vi "Format DescribeInstances_LVXML_ReservationSet_Loop.vi"(8 "error in (no error)":errorcluster, 11 "Siblings":T18(array[cluster])) -> (0 "error out":errorcluster, 3 "reservationSet":T1[](array[typedef]))   [LabVIEW 2014, in "AWS_EC2.lvlib" / "AWS_EC2.lvclass"]
uses:
  AWS_EC2.lvclass
  lv-xml-parser/r0/trunk/VI Source/EventType.ctl
  EC2 Datatypes/ReservationInfoType.ctl
  EC2 Datatypes/GroupItemType.ctl
  EC2 Datatypes/RunningInstancesItemsType.ctl
  EC2 Datatypes/InstanceStateType.ctl
  EC2 Datatypes/ProductCodeSetItemType.ctl
  EC2 Datatypes/PlacementResponseType.ctl
  EC2 Datatypes/GroupItemTypeSet.ctl
  EC2 Datatypes/StateReasonType.ctl
  EC2 Datatypes/InstanceBlockDeviceMappingResponseItemType.ctl
  EC2 Datatypes/EbsInstanceBlockDeviceMappingResponseType.ctl
  EC2 Datatypes/ResourceTagSetItemType.ctl
  EC2 Datatypes/InstanceNetworkInterfaceSetItemType.ctl
  EC2 Datatypes/InstanceNetworkInterfaceAttachmentType.ctl
  EC2 Datatypes/InstanceNetworkInterfaceAssociationType.ctl
  EC2 Datatypes/InstancePrivateIpAddressesSetItemType.ctl
  EC2 Datatypes/IamInstanceProfileResponseType.ctl
  lv-xml-parser/r0/trunk/VI Source/LV XML Parser.lvlib
  AWS_EC2.lvlib
panel:
  out "AWS_EC2 out":refnum<class "AWS_EC2.lvclass">
  in  "AWS_EC2 in":refnum<class "AWS_EC2.lvclass">
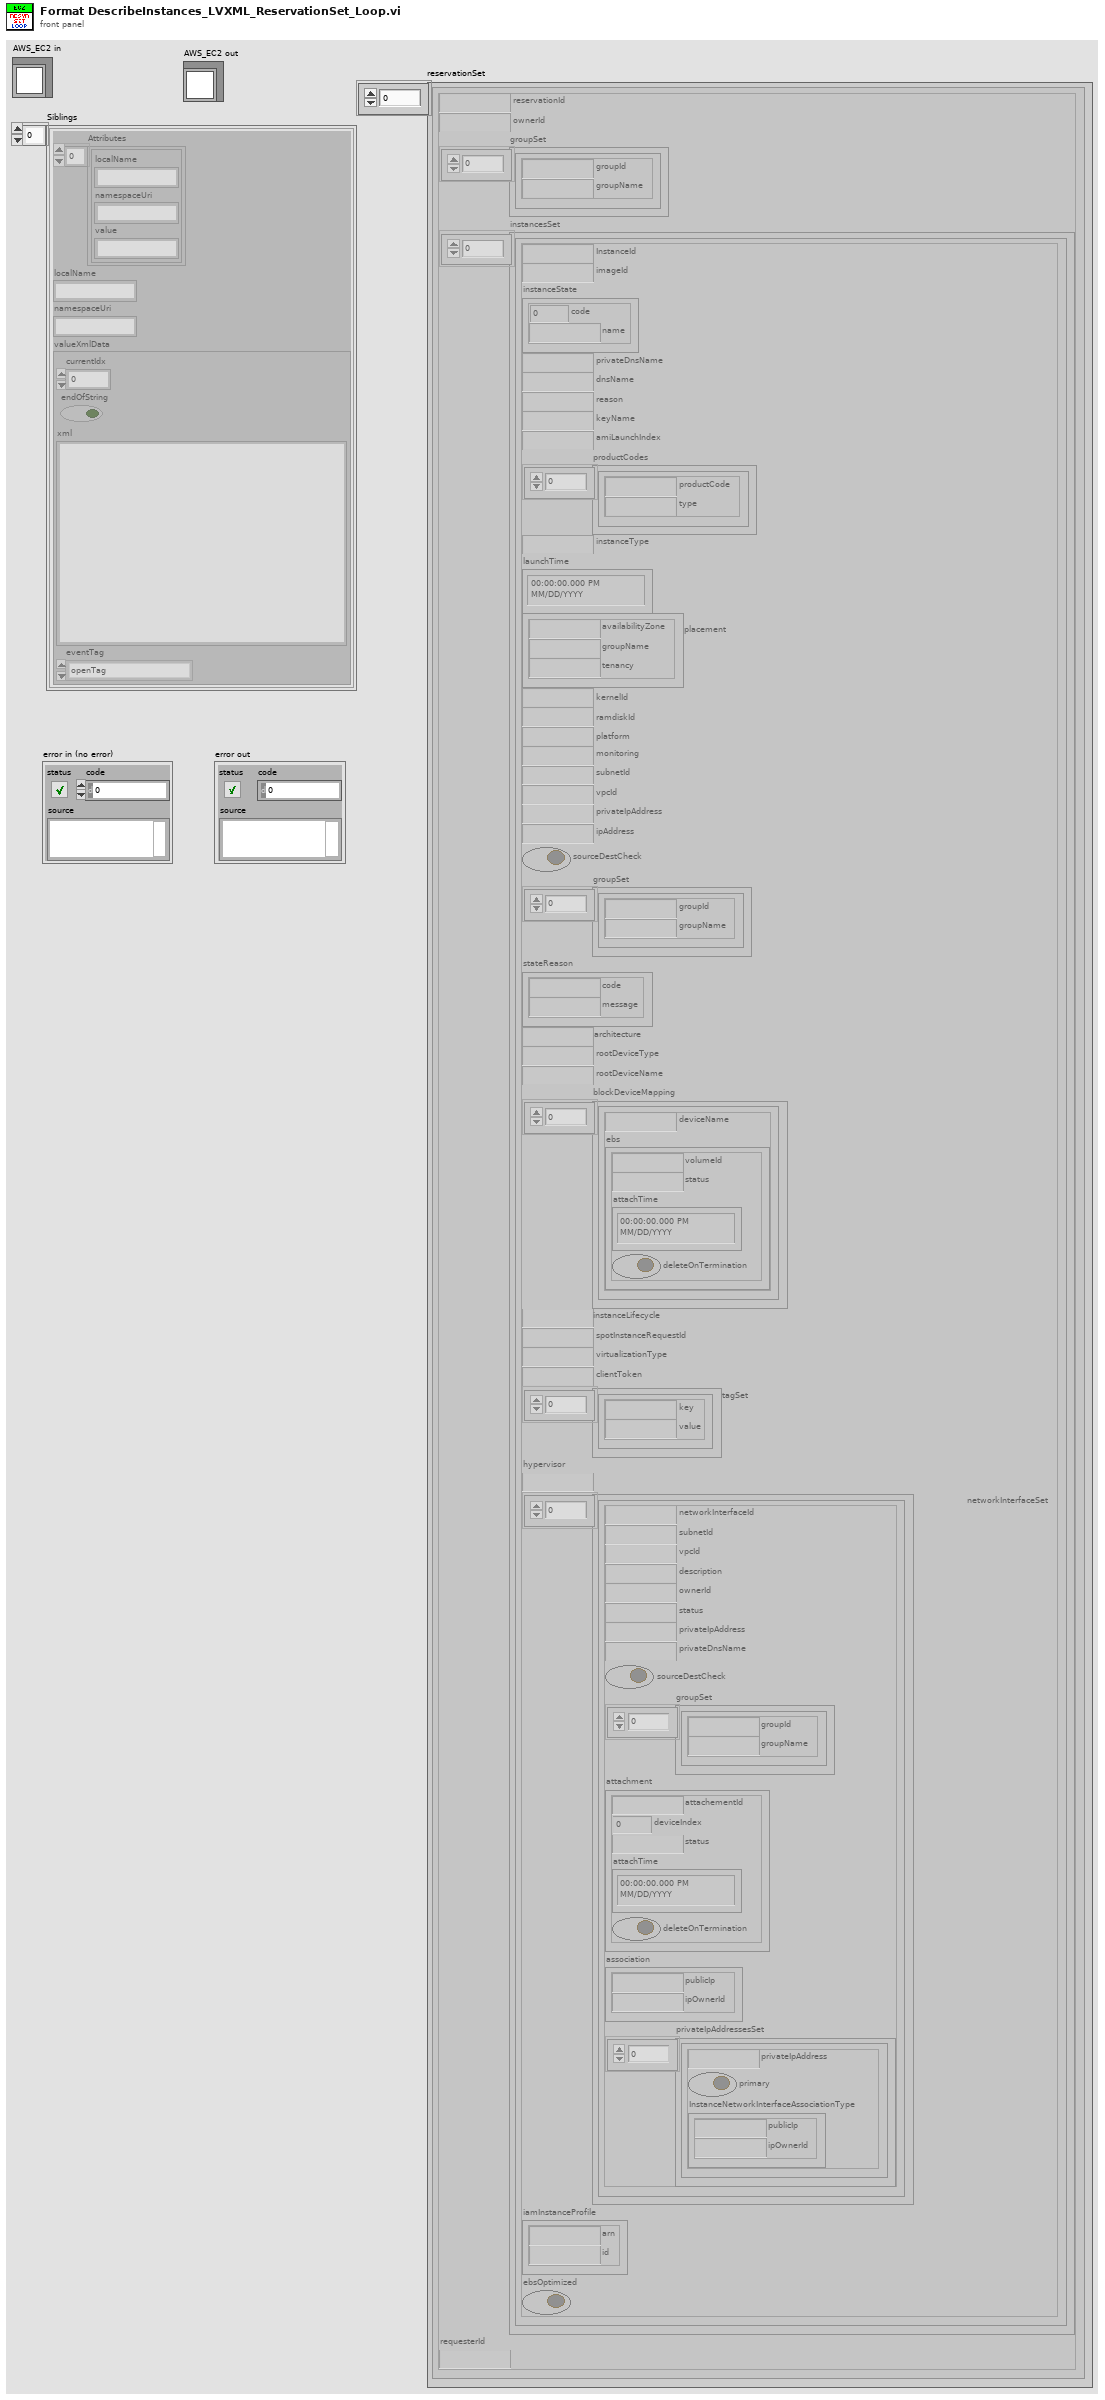
[diagram p1: front panel]
types:
  T1 = typedef "AWS_EC2.lvlib/ReservationInfoType.ctl" = cluster{"reservationId":string, "ownerId":string, "groupSet":T2[], "instancesSet":T3[], "requesterId":string}
  T2 = typedef "AWS_EC2.lvlib/GroupItemType.ctl" = cluster{"groupId":string, "groupName":string}
  T3 = typedef "AWS_EC2.lvlib/RunningInstancesItemsType.ctl" = cluster{"InstanceId":string, "imageId":string, "instanceState":T4, "privateDnsName":string, "dnsName":string, "reason":string, "keyName":string, "amiLaunchIndex":string, "productCodes":T5[], "instanceType":string, "launchTime":timestamp, "placement":T6, "kernelId":string, "ramdiskId":string, "platform":string, "monitoring":string, "subnetId":string, "vpcId":string, "privateIpAddress":string, "ipAddress":string, "sourceDestCheck":bool, "groupSet":T7, "stateReason":T8, "architecture":string, "rootDeviceType":string, "rootDeviceName":string, "blockDeviceMapping":T9[], "instanceLifecycle":string, "spotInstanceRequestId":string, "virtualizationType":string, "clientToken":string, "tagSet":T11[], "hypervisor":string, "networkInterfaceSet":T12[], "iamInstanceProfile":T16, "ebsOptimized":bool}
  T4 = typedef "AWS_EC2.lvlib/InstanceStateType.ctl" = cluster{"code":i16, "name":string}
  T5 = typedef "AWS_EC2.lvlib/ProductCodeSetItemType.ctl" = cluster{"productCode":string, "type":string}
  T6 = typedef "AWS_EC2.lvlib/PlacementResponseType.ctl" = cluster{"availabilityZone":string, "groupName":string, "tenancy":string}
  T7 = typedef "AWS_EC2.lvlib/GroupItemTypeSet.ctl" = T2[]
  T8 = typedef "AWS_EC2.lvlib/StateReasonType.ctl" = cluster{"code":string, "message":string}
  T9 = typedef "AWS_EC2.lvlib/InstanceBlockDeviceMappingResponseItemType.ctl" = cluster{"deviceName":string, "ebs":T10}
  T10 = typedef "AWS_EC2.lvlib/EbsInstanceBlockDeviceMappingResponseType.ctl" = cluster{"volumeId":string, "status":string, "attachTime":timestamp, "deleteOnTermination":bool}
  T11 = typedef "AWS_EC2.lvlib/ResourceTagSetItemType.ctl" = cluster{"key":string, "value":string}
  T12 = typedef "AWS_EC2.lvlib/InstanceNetworkInterfaceSetItemType.ctl" = cluster{"networkInterfaceId":string, "subnetId":string, "vpcId":string, "description":string, "ownerId":string, "status":string, "privateIpAddress":string, "privateDnsName":string, "sourceDestCheck":bool, "groupSet":T7, "attachment":T13, "association":T14, "privateIpAddressesSet":T15[]}
  T13 = typedef "AWS_EC2.lvlib/InstanceNetworkInterfaceAttachmentType.ctl" = cluster{"attachementId":string, "deviceIndex":i32, "status":string, "attachTime":timestamp, "deleteOnTermination":bool}
  T14 = typedef "AWS_EC2.lvlib/InstanceNetworkInterfaceAssociationType.ctl" = cluster{"publicIp":string, "ipOwnerId":string}
  T15 = typedef "AWS_EC2.lvlib/InstancePrivateIpAddressesSetItemType.ctl" = cluster{"privateIpAddress":string, "primary":bool, "InstanceNetworkInterfaceAssociationType":T14}
  T16 = typedef "AWS_EC2.lvlib/IamInstanceProfileResponseType.ctl" = cluster{"arn":string, "id":string}
  T17 = typedef "LV XML Parser.lvlib/EventType.ctl" = enum16{"openTag", "endOpenTag", "closeTag", "comment", "endComment", "endOfFile", "attribute", "startXml", "selfClosingTag"}
  T18 = cluster{"Attributes":cluster{"localName":string, "namespaceUri":string, "value":string}[], "localName":string, "namespaceUri":string, "valueXmlData":cluster{"currentIdx":i32, "endOfString":bool, "xml":string, "eventTag":T17}}[]
  T19 = cluster{"Attributes":cluster{"localName":string, "namespaceUri":string, "value":string}[], "localName":string, "namespaceUri":string, "valueXmlData":cluster{"currentIdx":i32, "endOfString":bool, "xml":string, "eventTag":T17}}
  T20 = cluster{"currentIdx":i32, "endOfString":bool, "xml":string, "eventTag":T17}
  T21 = cluster{"namespaceUri":string, "localName":string}
  T22 = cluster{"Attributes":cluster{"localName":string, "namespaceUri":string, "value":string}[], "localName":string, "namespaceUri":string, "valueXmlData":cluster{"currentIdx":i64, "endOfString":bool, "xml":string, "eventTag":T17}}[]
  T23 = cluster{"currentIdx":i64, "endOfString":bool, "xml":string, "eventTag":T17}
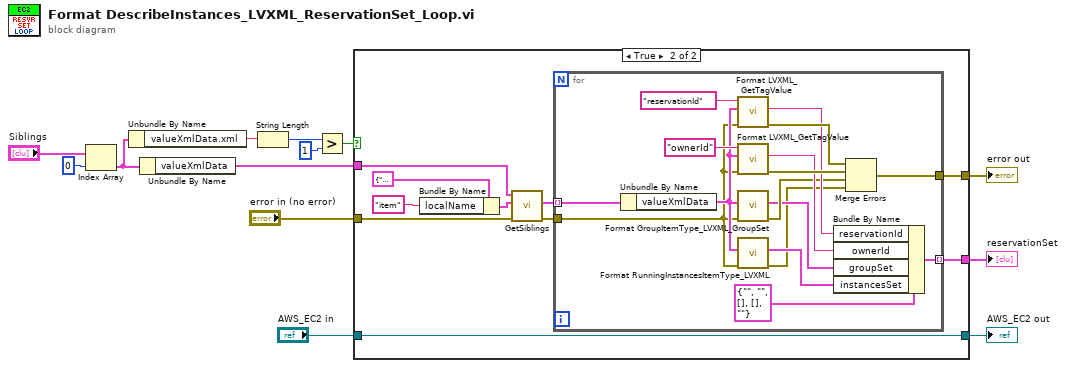
[diagram p0: block diagram]
diagram:
  n1 = Index Array(array="Siblings", index=0) -> (element=w12:T19)
  n2 = Unbundle By Name(w12) -> ("valueXmlData.xml"=w11:string)
  n3 = Unbundle By Name(w12) -> ("valueXmlData"=w10:T20)
  n4 = String Length(string=w11) -> (length=w7:i32)
  n5 = Greater?(x=w7, y=1) -> (0:w9:bool)
  n6 = case shown="True" w9 {
    tunnel: [w15 w24] -> w13
    tunnel: [_ w23] -> w3
    tunnel: "error in (no error)" -> [w15 w18]
    tunnel: w10 -> [_ w17]
    tunnel: "AWS_EC2 in" -> [w14 w16]
    tunnel: [w14 w16] -> w1
    frame False {
    }
    frame True {
      n7 = Bundle By Name(cluster=T21 {"namespaceUri"="", "localName"=""} ("limitToTag"), "localName"="item" ("Tag name")) -> (w20:T21)
      n8 = call "GetSiblings.vi"("error in (no error)"=w18, "limitToTag"=w20, "xmlData"=w17) -> ("error out"=w25:errorcluster, "Siblings"=w21:T22)  [unwired: 7 in]
      n9 = for {
        tunnel: w21 -> [w41] mode=indexing
        tunnel: [w34] -> w23 mode=indexing
        tunnel: [w40] -> w24
        tunnel: w25 -> [w27]
        n10 = Unbundle By Name(w41) -> ("valueXmlData"=w28:T23)
        n11 = call "Format LVXML_GetTagValue.vi"("error in (no error)"=w27, "xmlDataIn"=w28, "Tag name"="reservationId") -> ("error out"=w38:errorcluster, "Value"=w33:string)  [unwired: 6 in, 1 out]
        n12 = call "Format LVXML_GetTagValue.vi"("error in (no error)"=w27, "xmlDataIn"=w28, "Tag name"="ownerId") -> ("error out"=w39:errorcluster, "Value"=w32:string)  [unwired: 6 in, 1 out]
        n13 = call "Format GroupItemType_LVXML_GroupSet.vi"("error in (no error)"=w27, "valueXmlData"=w28) -> ("error out"=w31:errorcluster, "Array"=w30:T2[])  [unwired: 7 in, 1 out]
        n14 = call "Format RunningInstancesItemType_LVXML.vi"("error in (no error)"=w27, "valueXmlData"=w28) -> ("error out"=w26:errorcluster, "Array"=w29:T3[])  [unwired: 7 in, 1 out]
        n15 = Bundle By Name(cluster=T1 {"reservationId"="", "ownerId"="", "groupSet"=[], "instancesSet"=[], "requesterId"=""} ("ReservationInfoType"), "reservationId"=w33, "ownerId"=w32, "groupSet"=w30, "instancesSet"=w29) -> (w34:T1)
        n16 = Merge Errors(w38, w39, w31, w26) -> (w40:errorcluster)
      }
    }
  }
  "error out" <- w13
  "reservationSet" <- w3
  "AWS_EC2 out" <- w1
